vi "Preallocated A x Vector (DBL).vi"(9 "Preallocated A x vector":dbl[](array[numeric]) format="%.2f", 10 "Vector":dbl[](array[numeric]) format="%.2f", 11 "A":T1) -> (0 "error":i32, 3 "A x Vector":dbl[](array[numeric]) format="%.2f")   [LabVIEW 2020, in "NI_AALPro.lvlib"]
doc: "Performs the multiplication of two input matrices or an input matrix and an input vector. The data types you wire to the <B>A</B> and <B>B</B> inputs determine the polymorphic instance to use."
uses:
  NI_AALPro.lvlib
  RealMatrix.ctl
  <resource>/lvanlys.dll
  NI_Matrix.lvlib
panel:
  # "Preallocated A x Vector"
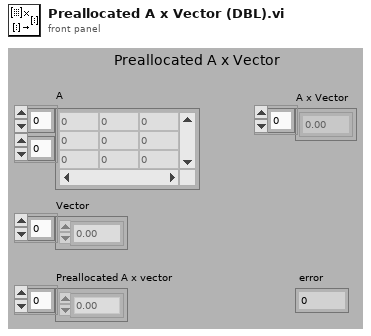
[diagram p1: front panel]
types:
  T1 = typedef "NI_Matrix.lvlib/RealMatrix.ctl" = dbl[][]
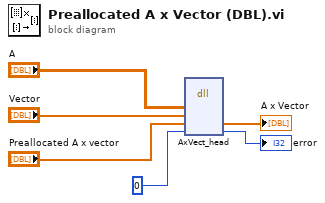
[diagram p0: block diagram]
diagram:
  n1 = dll-call lib="C:/Program Files (x86)/National Instruments/LabVIEW 2020/resource/lvanlys.*" fn="AxVect_head"("aHandle"="A", "xHandle"="Vector", "yHandle"="Preallocated A x vector", "dsperr"=0) -> ("yHandle"=→"A x Vector":dbl[], "dsperr"=→"error":i32)  [unwired: 6 in, 2 out]
